vi "Write Interlock_Enable.vi"(8 "error in":errorcluster, 10 "INTLK_Enable":bool, 11 "89XX in":refnum<class "89XX.lvclass">) -> (0 "error out":errorcluster, 3 "89XX out":refnum<class "89XX.lvclass">)   [LabVIEW 2019, in "89XX.lvlib" / "89XX.lvclass"]
uses:
  Library/89XX.lvclass
  C:/Users/Public/Documents/Development/builds/Engine/Monitored Actor.lvlibp/Monitored Actor/Monitored Actor/Monitored Actor.lvclass
  builds/Engine/Monitored Actor.lvlibp/Monitored Actor/Monitored Actor/Read Actor Label.vi
  builds/Instruments/PowerSupply.lvlibp/Library/PowerSupply.lvclass
  <vilib>/ErrorRing/Error Ring.xnode
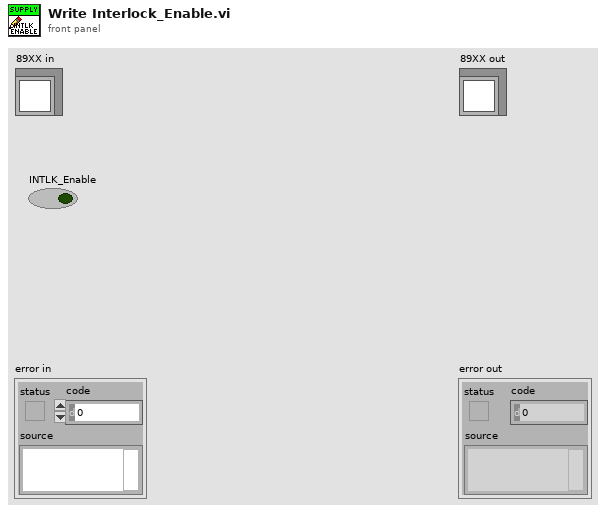
[diagram p1: front panel]
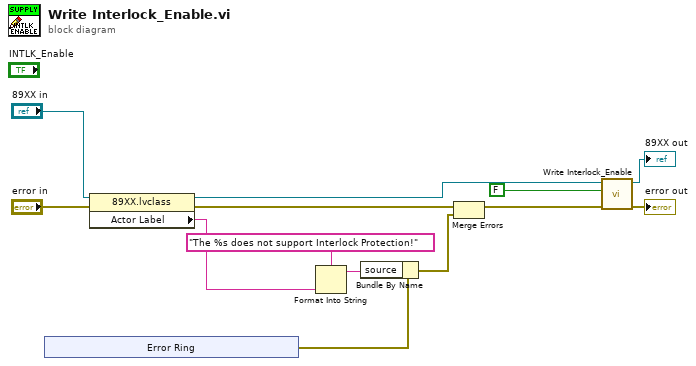
[diagram p0: block diagram]
diagram:
  n1 = xnode "Error Ring"() -> ("error out"=w7:errorcluster)
  n2 = property class="89XX.lvclass"(reference="89XX in", error in="error in") -> (reference out=w3:refnum<class "89XX.lvclass">, error out=w6:errorcluster, "Actor Label"=w10:string)
  n3 = Format Into String(format string="The %s does not support Interlock Protection!", w10) -> (resulting string=w8:string)  [unwired: 2 in, 1 out]
  n4 = Bundle By Name(cluster=w7, "source"=w8) -> (w9:errorcluster)
  n5 = Merge Errors(w6, w9) -> (w2:errorcluster)
  n6 = call-parent "Write Interlock_Enable.vi"("error in"=w2, "INTLK_Enable"=FALSE, "PowerSupply in"=w3) -> ("error out"=→"error out":errorcluster, "PowerSupply out"=→"89XX out":refnum<class "89XX.lvclass">)  [unwired: 7 in]
